vi "Flatten to ProjFile GObject Entry.vi"(8 "error in (no error)":errorcluster, 11 "GObject in":refnum<class "GObject.lvclass">) -> (0 "error out":errorcluster, 2 "GObject Data":T1, 3 "GObject out":refnum<class "GObject.lvclass">)   [LabVIEW 2013, in "SET Project Data.lvlib" / "GObject.lvclass"]
uses:
  GObject.lvclass
  Types/ProjFile_GObject Data.ctl
  GObject.lvclass/GObject.ctl
  SET Project Data.lvlib
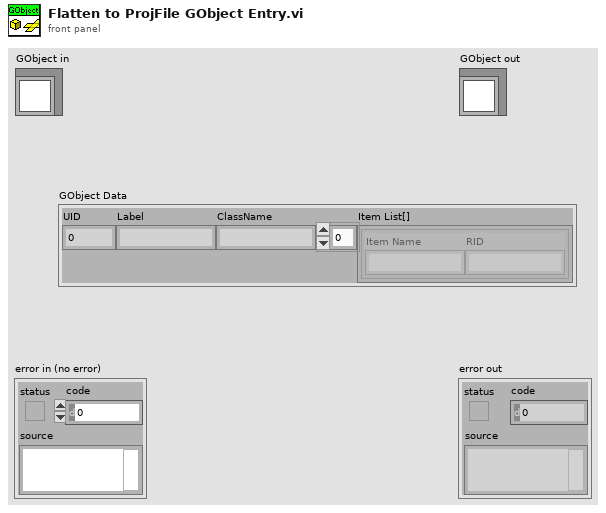
[diagram p1: front panel]
types:
  T1 = typedef "SET Project Data.lvlib/ProjFile_GObject Data.ctl" = cluster{"UID":i32, "Label":string, "ClassName":string, "Item List[]":cluster{"Item Name":string, "RID":string}[]}
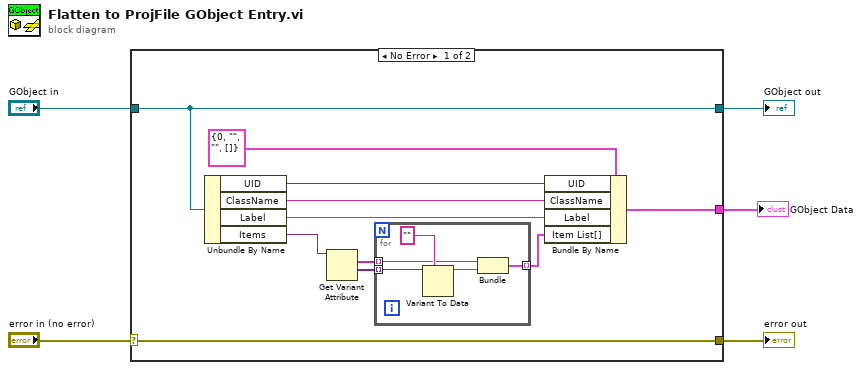
[diagram p0: block diagram]
diagram:
  n1 = case shown="No Error" "error in (no error)" {
    selector: "error in (no error)" -> [w16 w23]
    tunnel: [w16 w23] -> w4
    tunnel: [w15 w22] -> w2
    tunnel: "GObject in" -> [w15 w22]
    tunnel: [w6 _] -> w1
    frame No Error {
      n2 = Unbundle By Name(w15) -> ("UID"=w10:i32, "ClassName"=w9:string, "Label"=w8:string, "Items"=w14:variant)
      n3 = Get Variant Attribute(Variant=w14) -> (names=w13:string[], values=w12:variant[])  [unwired: 3 in, 2 out]
      n4 = for {
        tunnel: w13 -> [w18] mode=indexing
        tunnel: w12 -> [w21] mode=indexing
        tunnel: [w17] -> w7 mode=indexing
        n5 = Variant To Data(type="", Variant=w21) -> (data=w19:string)  [unwired: 1 in, 1 out]
        n6 = Bundle(w18, w19) -> (w17:cluster{string, string})  [unwired: 1 in]
      }
      n7 = Bundle By Name(cluster=T1 {"UID"=0, "Label"="", "ClassName"="", "Item List[]"=[]} ("GObject Data"), "UID"=w10, "ClassName"=w9, "Label"=w8, "Item List[]"=w7) -> (w6:T1)
    }
    frame Error {
    }
  }
  "error out" <- w4
  "GObject out" <- w2
  "GObject Data" <- w1
